vi "CO Serial CAL & Data Recording & DECADEv4.0.vi"() -> ()   [LabVIEW 2014]
uses:
  <vilib>/Platform/TimedLoop/XDataNode/timing_clust.ctl
  <vilib>/Platform/TimedLoop/XDataNode/nitl_modes.ctl
  <vilib>/Platform/TimedLoop/XDataNode/wakeup.ctl
  C:/Program Files (x86)/National Instruments/LabVIEW 2014/examples/Data Communication/Network Streams/Simple Network Streams/support/Network Stream Command.ctl
  <vilib>/Utility/error.llb/whitespace.ctl
  <vilib>/Instr/_visa.llb/VISA Configure Serial Port (Instr).vi
  <vilib>/Utility/tcp.llb/UDP Multicast Write-Only Open.vi
  <vilib>/platform/TimedLoop/XDataNode/XDataNode.xnode
  <vilib>/Platform/TimedLoop/XDataNode/XDNodeRunTimeDep.lvlib
panel:
  out "Stop File Write":bool
  out "Default file name":string
  in  "Flight Number 2":string="XXXX"
  out "status":bool
  out "CO Vacuum":bool
  out "CO CAL":bool
  out "error out":errorcluster
  out "CO Vacuum?":i16
  out "Control data":i32[](array[numeric])
  out "Control data out":string
  in  "VISA resource name":refnum<visa-resource-name>="ASRL8::INSTR"
  out "Serial VISA error":errorcluster
  out "SEPTIC TCP Error Out":errorcluster
  out "TCP packet\nSend To SEPTIC":bool
  in  "msec to wait":u32=330 caption="mSec to Wait"
  out "UDP Time Stamp Offset":i32=1
  out "Scan from String Error \nCounter from process loop":i32
  out "TCP Binary Packet":string
  in  "ue9LJ temp":u16
  out "FISH TCP Error Out":errorcluster
  out "TCP packet\nSend To FISH":bool
  out "UDP_Out_Error Out":errorcluster
  out "Data Array":string[](array[string])
  out "UDP_Out Status":bool
  out "Data Process Status":bool
  out "Command In":string[](array[string])
  out "ERR Counter":i32
  out "UDP_Out":string
  out "UDP_Pack_num":u32
  out "Flight Number":string
  out "OK RAW COUNTER":i32
  out "IN_CAL?":bool
  out "Redundent DATA":string
  out "Data String":string
  out "CO_Data_Buffer":string[](array[string])
  out "RAW DATA":string
  out "loop count":i32
  out "Number of Read error":i32
  out "Command In":string
  # "Pre-flight"
  # "CONC"
  # "SIG"
  # "SENS"
  # "ZERO"
  # "Lamp flow controller"
  # "Lamp temperature"
  # "Monochromater flow controller"
  # "Monochromater temperature"
  # "Monochromater pressure"
  # "Fluorescence cell pressure"
  # "Calibration gas pressure"
  # "Cell temperature"
  # "Calibration Concentration"
  # "ERROR number"
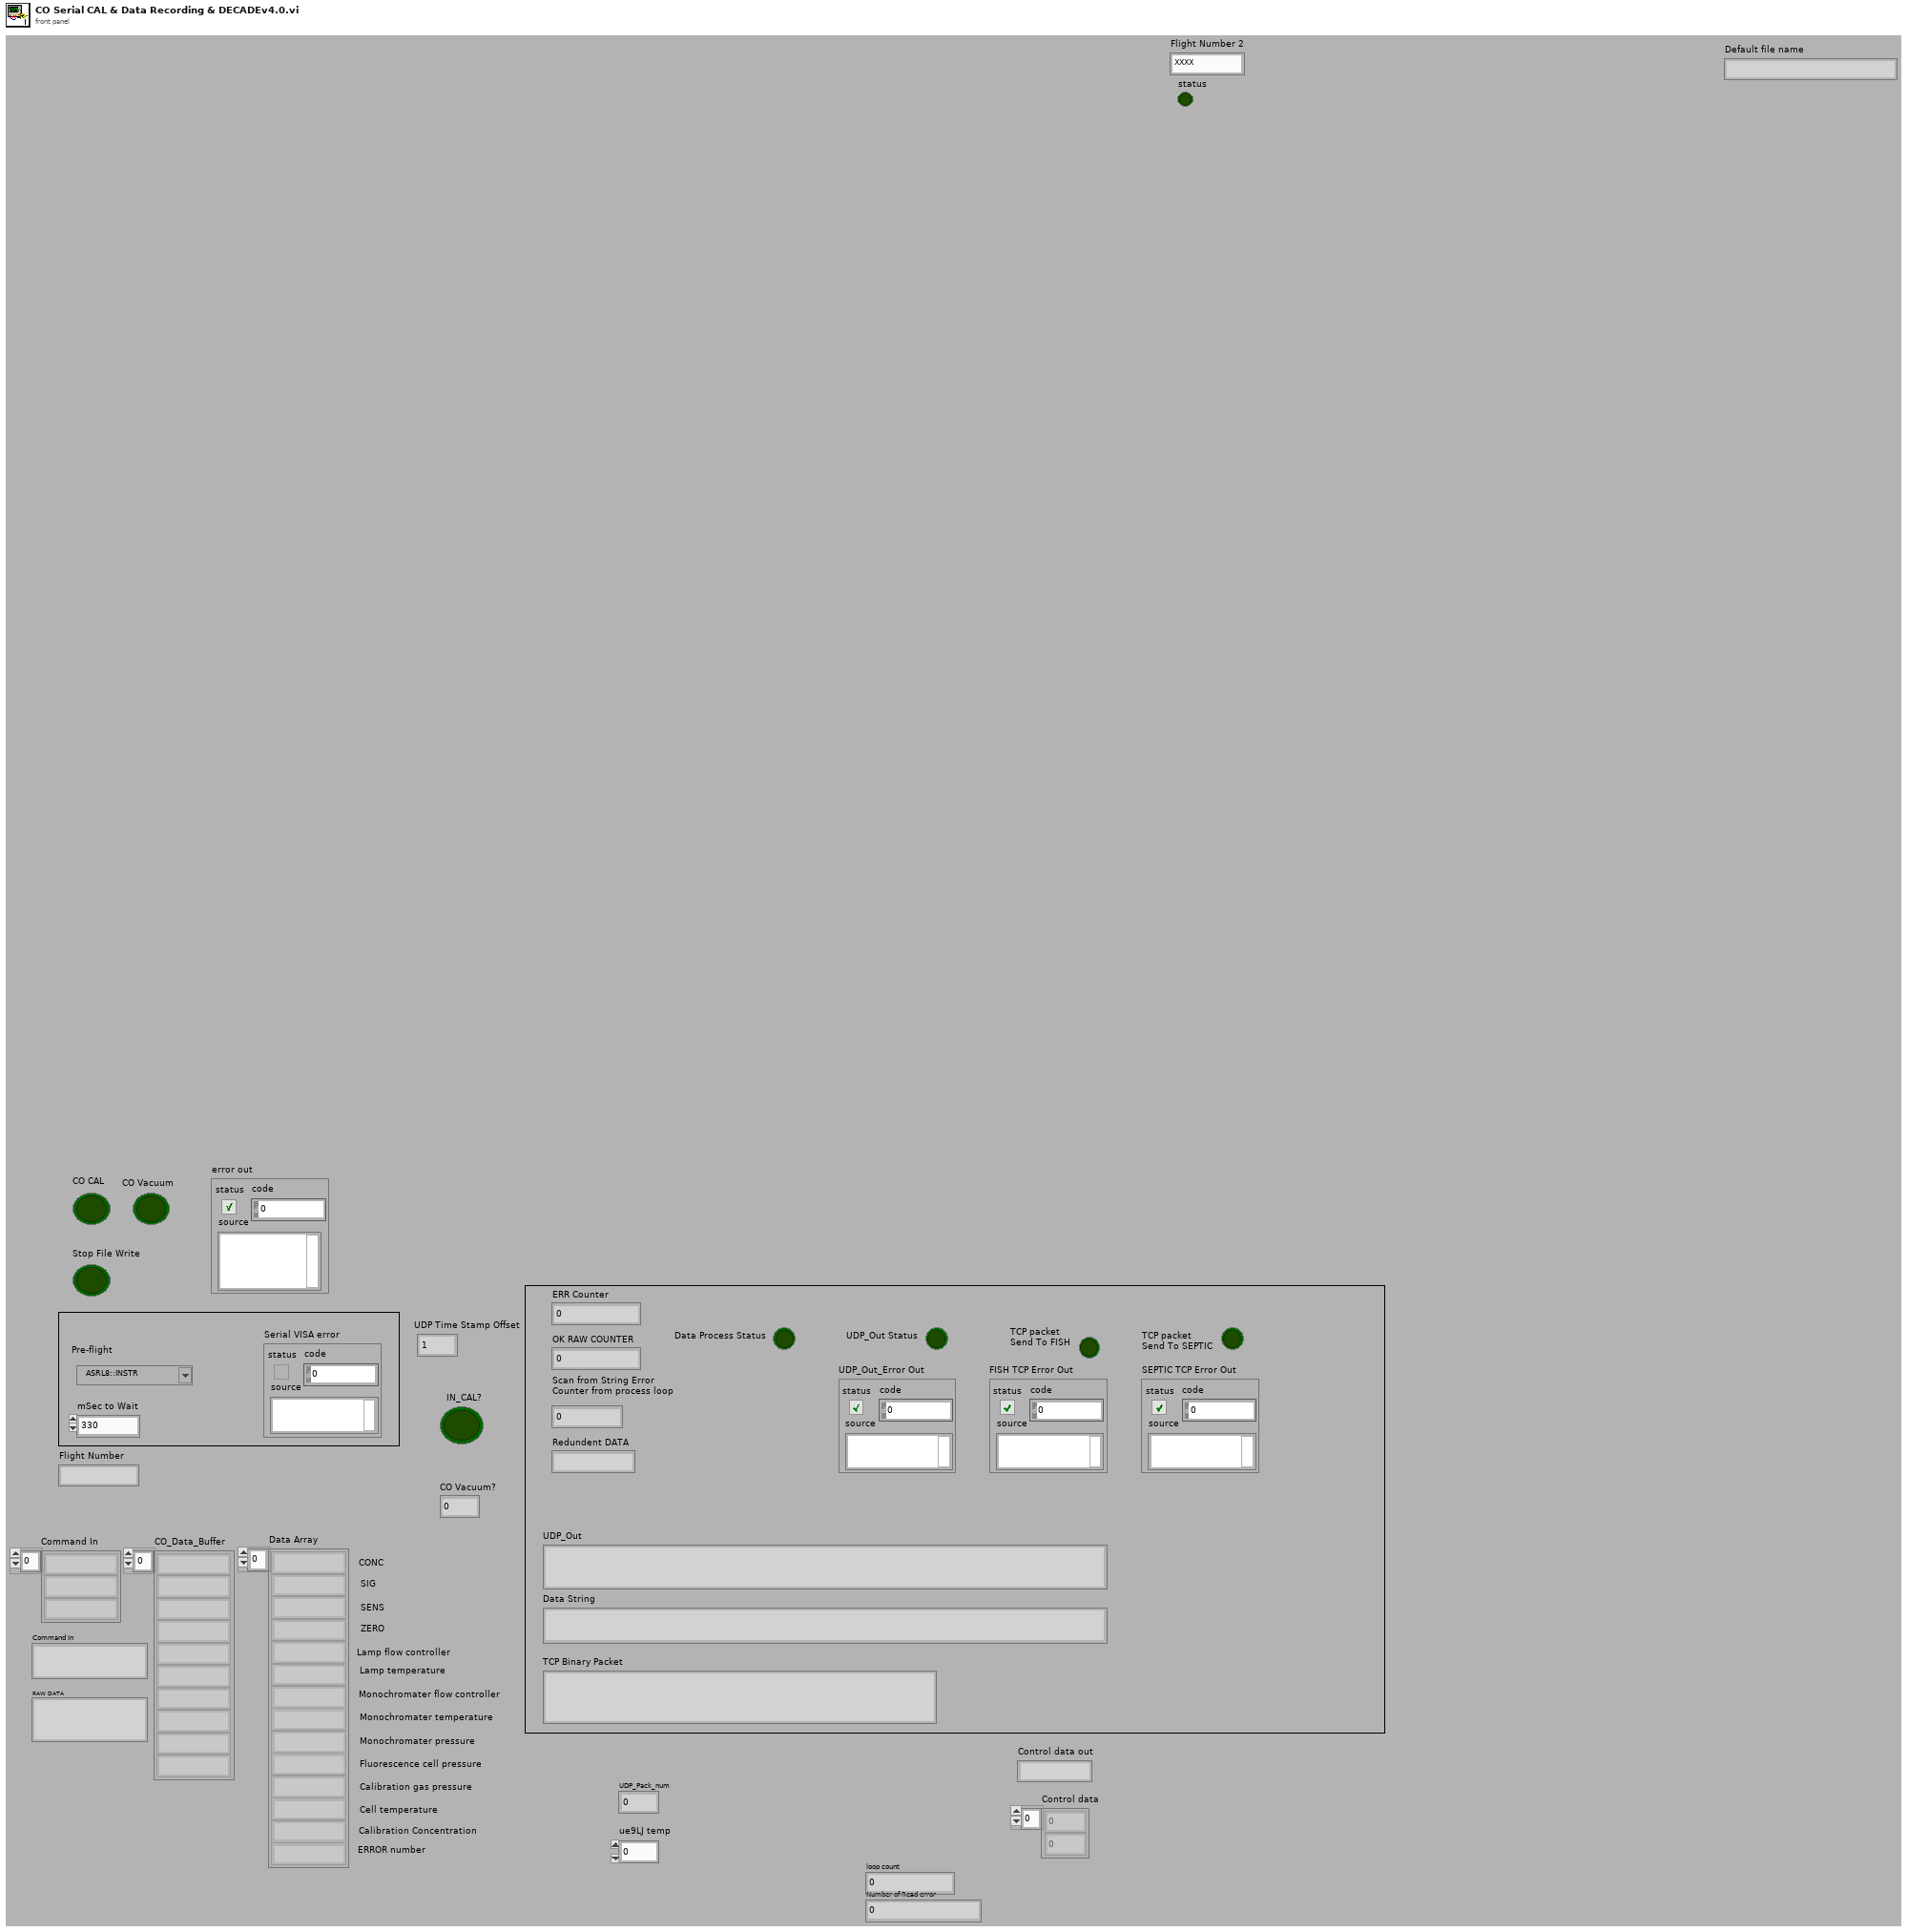
[diagram p1: front panel]
types:
  T1 = typedef "XDNodeRunTimeDep.lvlib/timing_clust.ctl" = cluster{"Expected End [f-1]":u64, "Actual End [f-1]":u64, "Finished Late? [f-1]":bool, "Expected End [i-1]":u64, "Actual End [i-1]":u64, "Finished Late? [i-1]":bool, "Expected Start [i]":u64, "Actual Start [i]":u64, "Expected Start [f]":u64, "Actual Start [f]":u64, "Source Name":string, "Structure Name":string, "Period":i64, "Deadline":i64, "Offset":i64, "Start":i64, "Priority":i32, "Timeout":i32, "Mode":T2, "Wakeup Reason":T3, "Error":errorcluster, "Source Type":string, "Secondary Source Type":string, "Global End Time":u64, "Global Start Time":u64, "Frame Duration":u64, "Iteration Duration":u64, "Assigned CPU":i32, "I/O Scan Engine Mode":u32}
  T2 = typedef "XDNodeRunTimeDep.lvlib/nitl_modes.ctl" = enum32{"No Change", "Process missed periods, maintain original phase", "Discard missed periods, maintain original phase", "Process missed periods, ignore original phase", "Discard missed periods, ignore original phase"}
  T3 = typedef "XDNodeRunTimeDep.lvlib/wakeup.ctl" = enum32{"Normal", "Aborted", "Asynchronous wakeup", "Timing source error", "Timed loop error", "Timeout"}
  T4 = typedef "Network Stream Command.ctl" = cluster{"Message":string, "Message Data":variant}
  T5 = enum16{"open", "replace", "create", "open or create", "replace or create", "replace or create with confirmation"}
  T6 = typedef "whitespace.ctl" = u16
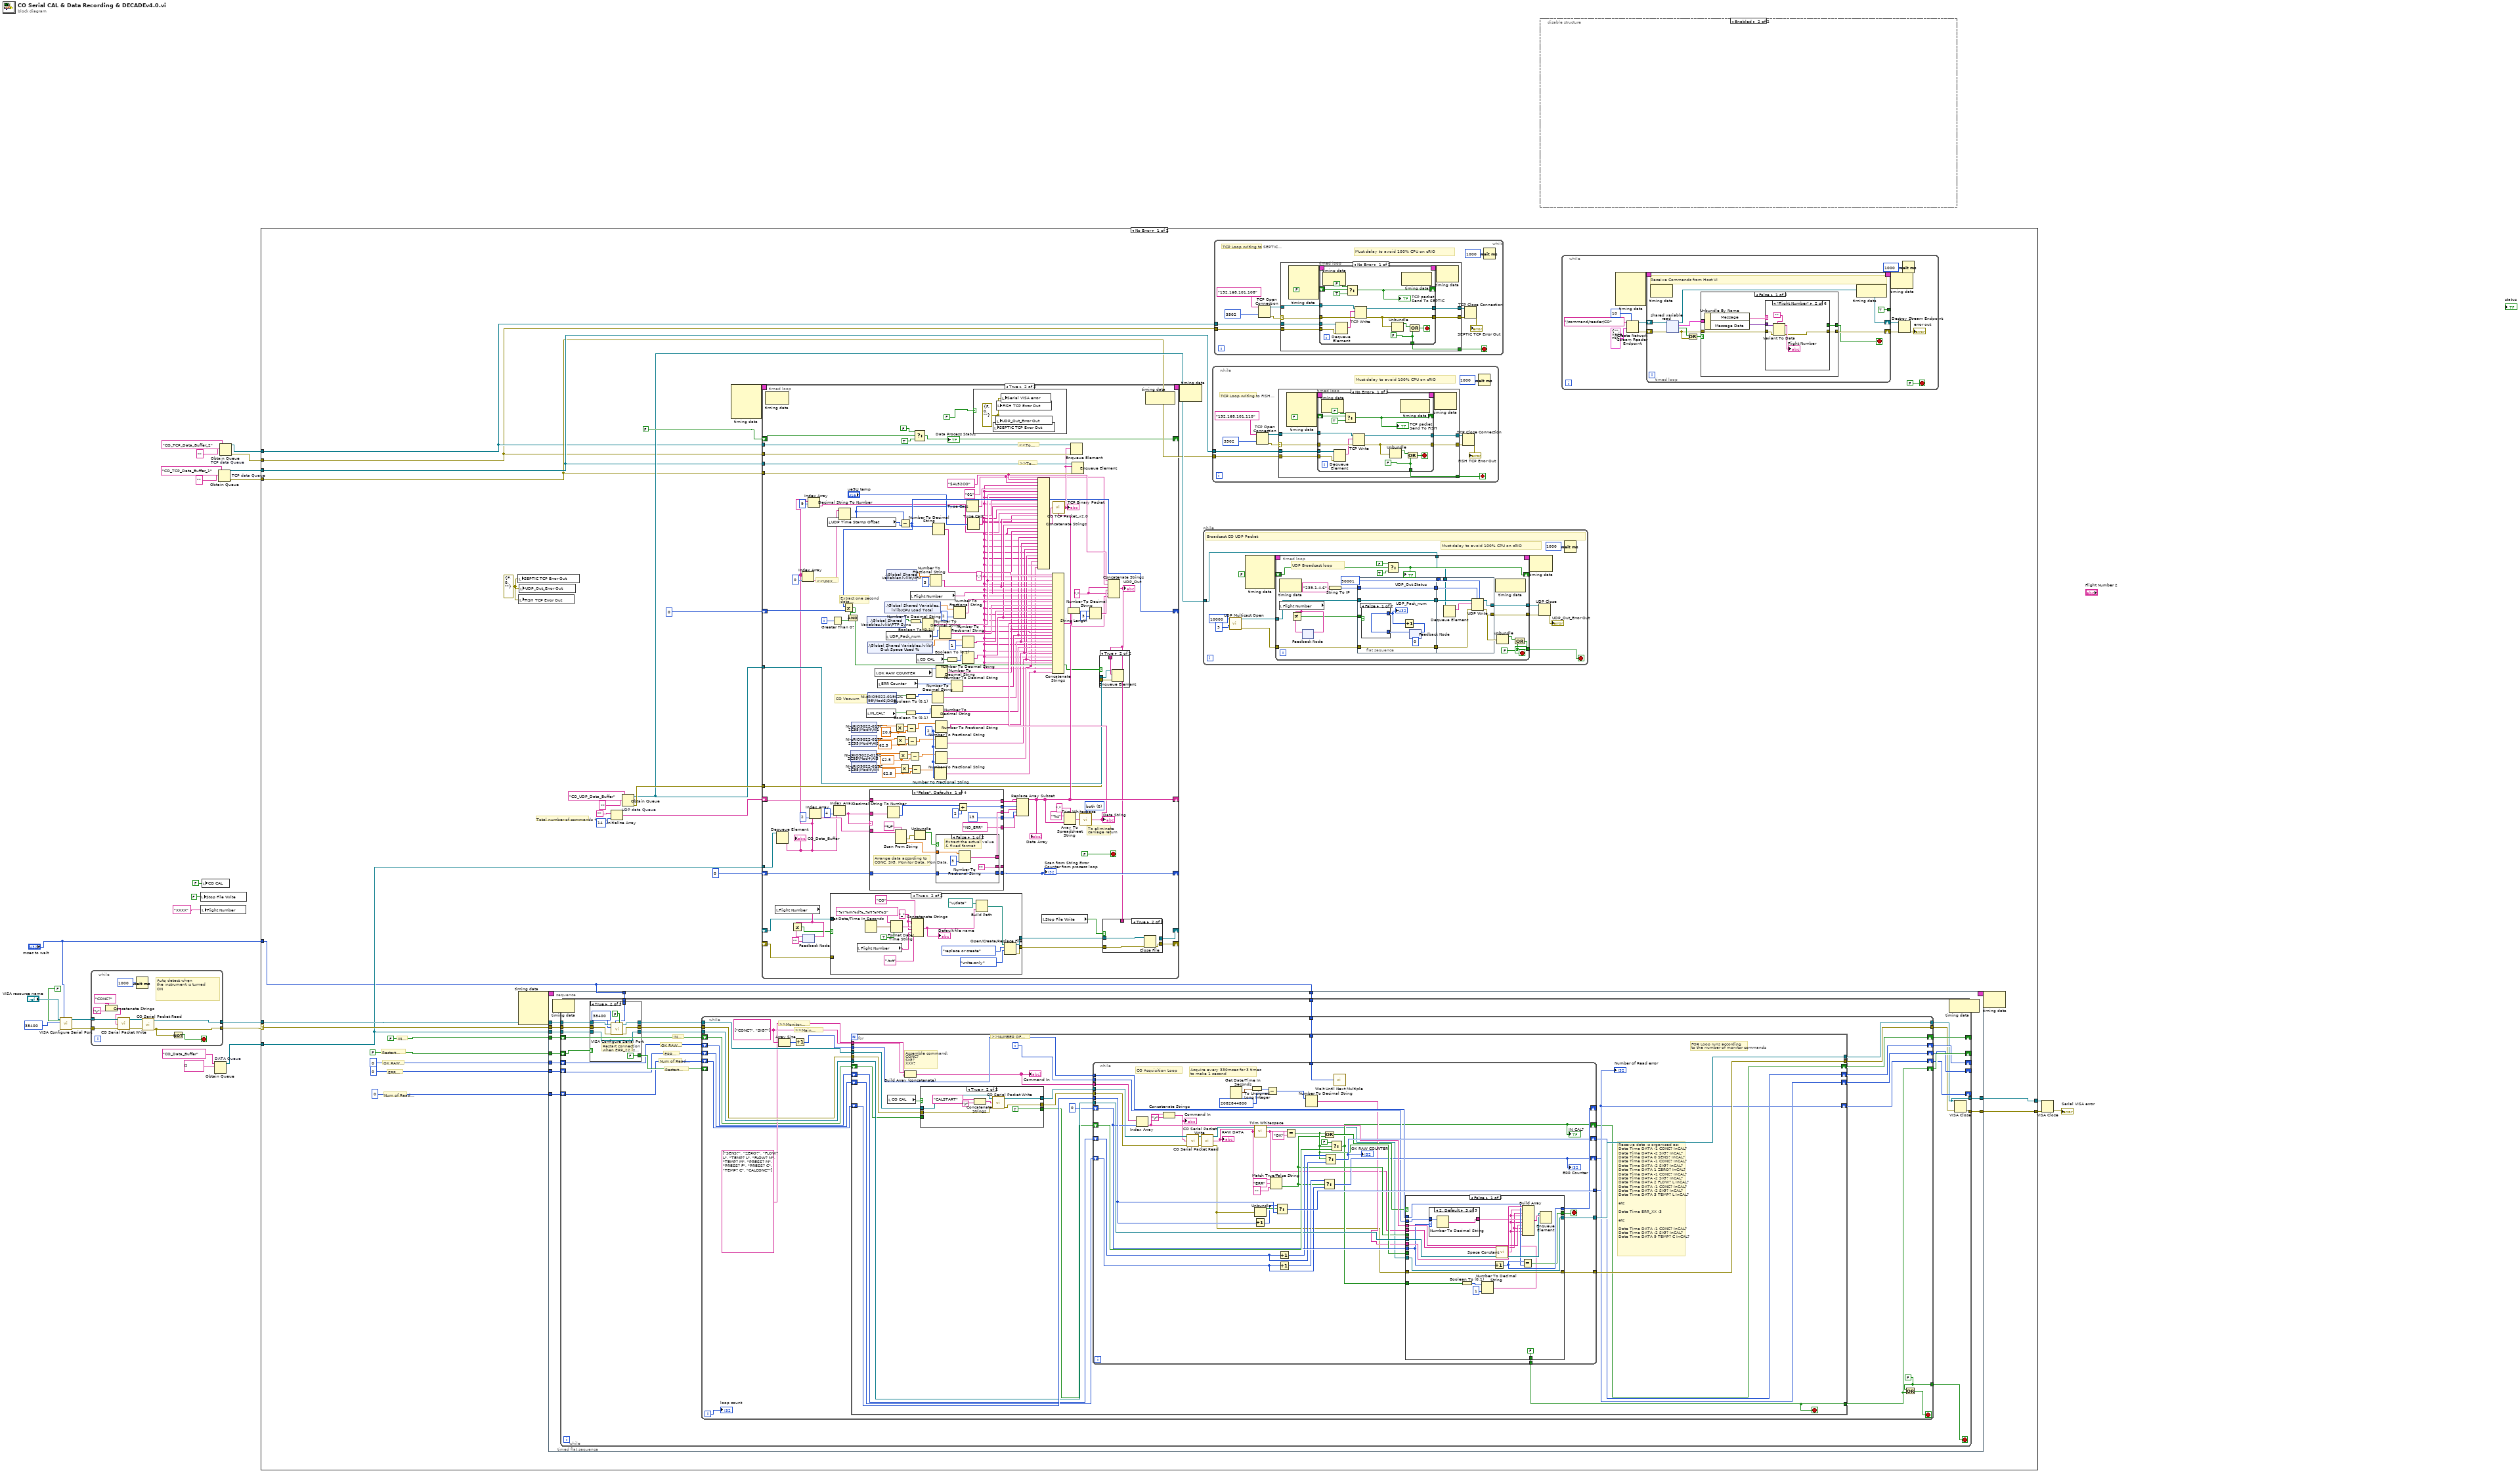
[diagram p0: block diagram]
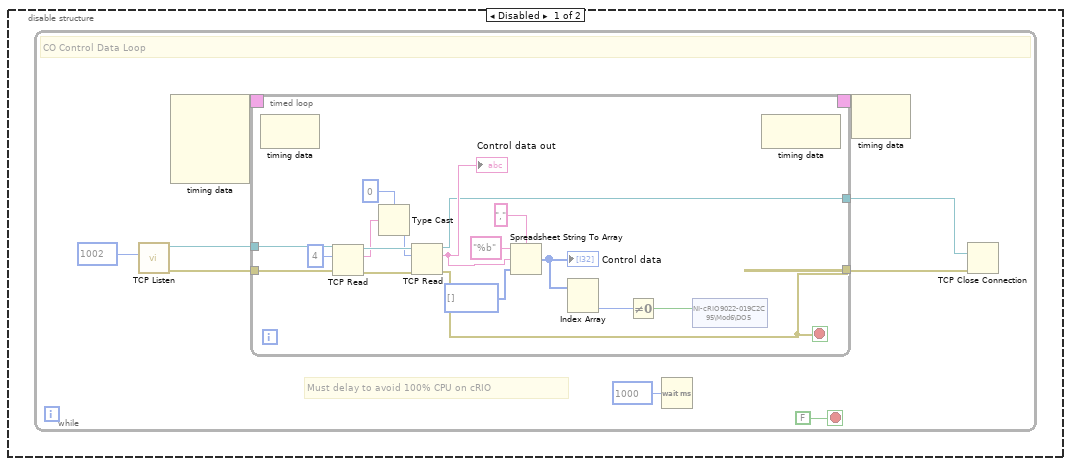
[diagram p2: hidden frame]
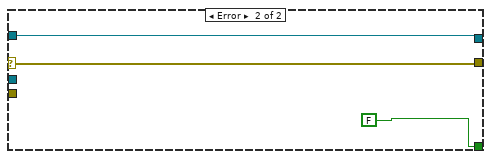
[diagram p3: hidden frame]
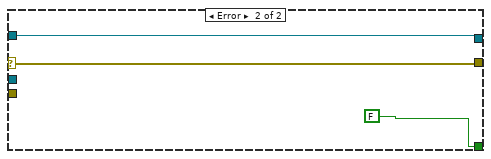
[diagram p4: hidden frame]
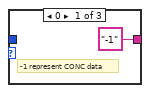
[diagram p6: hidden frame]
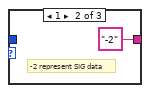
[diagram p7: hidden frame]
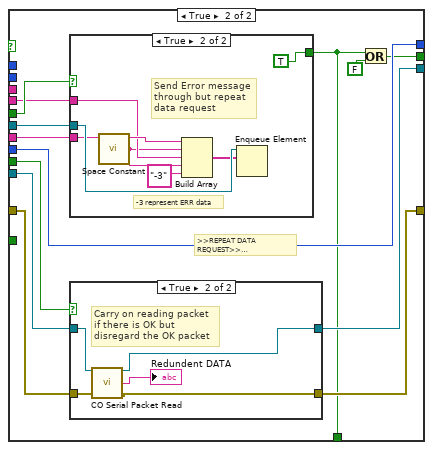
[diagram p8: hidden frame]
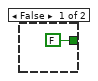
[diagram p10: hidden frame]
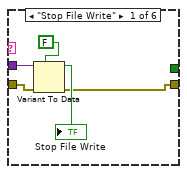
[diagram p12: hidden frame]
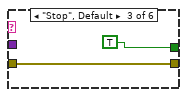
[diagram p13: hidden frame]
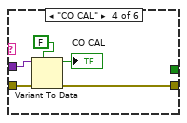
[diagram p14: hidden frame]
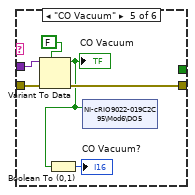
[diagram p15: hidden frame]
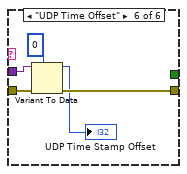
[diagram p16: hidden frame]
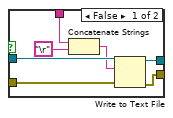
[diagram p19: hidden frame]
diagram:
  n1 = call-poly "VISA Configure Serial Port"("VISA resource name"="VISA resource name", "timeout (10sec)"="msec to wait", "Enable Termination\nChar (T)"=FALSE ("Enable Termination\nChar (T)"), "baud rate (9600)"=u32 38400) -> ("VISA resource name out"=w12:refnum<visa-resource-name>, "error out"=w11:errorcluster)  [unwired: 10 in]
  n2 = while {
    tunnel: w12 -> [w36]
    tunnel: w11 -> [w35]
    tunnel: [w29] -> w10
    tunnel: [w30] -> w9
    stop <- w34 stop-if-true
    # "Auto detect when\nthe instrument is turned \nON"
    n3 = Concatenate Strings("CONC?" ("Data in"), "\r") -> (w26:string)
    n4 = call "CO Serial Packet Write.vi"("VISA resource name In"=w36, "Data in"=w26, "error in (no error)"=w35) -> ("VISA resource name Out"=w32:refnum<visa-resource-name>, "error out"=w31:errorcluster)  [unwired: 11 in]
    n5 = Wait (ms)(milliseconds to wait=u32 1000) -> ()  [unwired: 1 out]
    n6 = call "CO Serial Packet Read.vi"("VISA resource In"=w32, "error in"=w31) -> ("VISA resource Out"=w29:refnum<visa-resource-name>, "error out"=w30:errorcluster)  [unwired: 11 in, 1 out]
    n7 = Not(x=w30) -> (.not. x?=w34:bool)
  }
  n8 = local write "Stop File Write"(FALSE ("Stop File Write")) -> ()
  n9 = local write "Flight Number"("XXXX" ("Flight Number")) -> ()
  n10 = local write "CO CAL"(FALSE ("CO CAL")) -> ()
  n11 = Obtain Queue "DATA Queue"(name (unnamed)="CO_Data_Buffer", element data type=string[] []) -> (queue out=w23:refnum<queue>)  [unwired: 3 in, 2 out]
  n12 = Obtain Queue "TCP data Queue"(name (unnamed)="CO_TCP_Data_Buffer_1", element data type="") -> (queue out=w22:refnum<queue>, error out=w21:errorcluster)  [unwired: 3 in, 1 out]
  n13 = Obtain Queue "TCP data Queue"(name (unnamed)="CO_TCP_Data_Buffer_2", element data type="") -> (queue out=w20:refnum<queue>, error out=w19:errorcluster)  [unwired: 3 in, 1 out]
  n14 = case shown="No Error" w9 {
    selector: w9 -> [w64 w717]
    tunnel: w10 -> [w65 w716]
    tunnel: [w66 w717] -> w15
    tunnel: [w42 w716] -> w14
    tunnel: w23 -> [w63 _]
    tunnel: w22 -> [w52 _]
    tunnel: w21 -> [w51 _]
    tunnel: w20 -> [w50 _]
    tunnel: w19 -> [w49 _]
    tunnel: "msec to wait" -> [w37 _]
    frame No Error {
      w48 = errorcluster {"status"=FALSE, "code"=0, "source"=""} ("UDP_Out_Error Out")
      # "Restart connection?"
      # "IN CAL?"
      # "OK RAW Counter"
      # "ERR Counter"
      # "Num of Read Error"
      # "Total number of commands + ERR"
      n15 = local write "SEPTIC TCP Error Out"(w48) -> ()
      n16 = node-c288() -> (w39:T1)  [unwired: 4 in]
      n17 = local write "FISH TCP Error Out"(w48) -> ()
      n18 = local write "UDP_Out_Error Out"(w48) -> ()
      n19 = timed-sequence {
        timing: w39 -> [_]
        timing-out: [_] -> w38
        tunnel: [w162] -> w66
        tunnel: w65 -> [w161]
        tunnel: w64 -> [w160]
        tunnel: w63 -> [w159]
        tunnel: FALSE -> [w158]
        tunnel: 0 -> [w157]
        tunnel: 0 -> [w156]
        tunnel: 0 -> [w155]
        tunnel: FALSE ("IN_CAL?") -> [w154]
        tunnel: [w153] -> w42
        tunnel: w37 -> [w152]
        tunnel: w37 -> [w151]
        n20 = timed-flat-sequence {
          tunnel: [w174] -> w162
          tunnel: w161 -> [w173]
          tunnel: w160 -> [w172]
          tunnel: w159 -> [w171]
          tunnel: w158 -> [w170]
          tunnel: w157 -> [w169]
          tunnel: w156 -> [w168]
          tunnel: w155 -> [w167]
          tunnel: w154 -> [w166]
          tunnel: [w165] -> w153
          tunnel: w152 -> [w164]
          tunnel: w151 -> [w163]
          n21 = node-c288() -> ()  [unwired: 1 in, 1 out]
          n22 = while {
            tunnel: [w179] -> w174
            tunnel: w173 -> [w196]
            tunnel: w172 -> [w195]
            tunnel: w171 -> [w193]
            shift-right: [w190] -> _
            shift-left: w170 -> [w191]
            shift-right: [w186] -> _
            shift-left: w169 -> [w187]
            shift-right: [w183] -> _
            shift-left: w168 -> [w185]
            shift-right: [w182] -> _
            shift-left: w167 -> [w184]
            shift-right: [w180] -> _
            shift-left: w166 -> [w181]
            tunnel: [w177] -> w165
            tunnel: w164 -> [w176]
            tunnel: w163 -> [w175]
            stop <- w189 stop-if-true
            # "Restart connection?"
            # "Num of Read Error"
            # "ERR Counter"
            # "IN CAL?"
            # "OK RAW Counter"
            n23 = case shown="True" w191 {
              selector: w191 -> [w198 _]
              tunnel: [w201 w207] -> w197
              tunnel: w196 -> [w201 w208]
              tunnel: [w200 w206] -> w194
              tunnel: w195 -> [w200 w205]
              tunnel: [w199 w210] -> w192
              tunnel: w193 -> [w199 w210]
              tunnel: [w198 FALSE] -> w188
              tunnel: w175 -> [_ w202]
              frame False {
              }
              frame True {
                # "Restart connection\nwhen ERR_22 is detected"
                n24 = call-poly "VISA Configure Serial Port"("VISA resource name"=w208, "timeout (10sec)"=w202, "Enable Termination\nChar (T)"=FALSE ("Enable Termination\nChar (T)"), "baud rate (9600)"=u32 38400, "error in (no error)"=w205) -> ("VISA resource name out"=w207:refnum<visa-resource-name>, "error out"=w206:errorcluster)  [unwired: 9 in]
              }
            }
            n25 = while {
              tunnel: [w232] -> w178
              tunnel: w197 -> [w231]
              tunnel: w194 -> [w230]
              tunnel: [w229] -> w177
              tunnel: w192 -> [w228]
              shift-right: [w219] -> w186
              shift-left: w187 -> [w223]
              shift-right: [w218] -> w183
              shift-left: w185 -> [w222]
              shift-right: [w217] -> w180
              shift-left: w181 -> [w221]
              shift-right: [w216] -> w182
              shift-left: w184 -> [w220]
              tunnel: [w212] -> w189
              shift-right: [w213] -> w190
              shift-left: w188 -> [_]
              tunnel: w176 -> [w211]
              i -> [w215]
              stop <- w214 stop-if-true
              w212 = FALSE
              w227 = string[] ["CONC?", "SIG?"]
              # ">>Main commands>>"
              # ">>Monitor Command>>"
              n26 = Array Size(array=w227) -> (size(s)=w224:i32)
              n27 = Increment(x=w224) -> (x+1=w226:i32)
              n28 = for {
                tunnel: w231 -> [w252]
                tunnel: w230 -> [w251]
                tunnel: [w257] -> w232
                shift-right: [w255] -> w216
                shift-left: w220 -> [w256]
                tunnel: [w254] -> w229
                tunnel: w228 -> [w253]
                tunnel: w226 -> [w247]
                shift-right: [w245] -> w217
                shift-left: w221 -> [w246]
                shift-right: [w243] -> w218
                shift-left: w222 -> [w244]
                shift-right: [w241] -> w219
                shift-left: w223 -> [w242]
                tunnel: string[] ["SENS?", "ZERO?", "FLOW? L", "TEMP? L", "FLOW? M", "TEMP? M", "PRESS? M", "PRESS? F", "PRESS? C", "TEMP? C", "CALCONC?"] -> [w238] mode=indexing
                tunnel: w227 -> [w239]
                tunnel: [w236] -> w213
                tunnel: w211 -> [w234]
                i -> [w237]
                stop <- w236 stop-if-true
                # "Receive data is organised as:\nDate Time DATA -1 CONC? InCAL?\nDate Time DATA -2 SIG? InCAL?\nDate Time DATA 0 SENS? InCAL?\nDate Time DATA -1 CONC? InCAL?\nDate Time DATA -2 SIG? InCAL?\nDate Time DATA 1 ZERO? InCAL?\nDate Time DATA -1 CONC? InCAL?\nDate Time DATA -2 SIG? InCAL?\nDate Time DATA 2 FLOW? L InCAL?\nDate Time DATA -1 CONC? InCAL?\nDate Time DATA -2 SIG? InCAL?\nDate Time DATA 3 TEMP? L InCAL?\n\netc\n\nDate Time ERR_XX -3\n\netc\n\nDate Time DATA -1 CONC? InCAL?\nDate Time DATA -2 SIG? InCAL?\nDate Time DATA 9 TEMP? C InCAL?"
                # "FOR Loop runs according\nto the number of monitor commands"
                # "Assemble command:\nCONC?\nSIG?\nXXX?"
                # ">>NUMBER OF COMMANDS>>"
                n29 = local read "CO CAL"() -> (w233:bool)
                n30 = Build Array (concatenate)(w239, w238) -> (w240:string[])
                "Command In" <- w240
                n31 = case shown="True" w233 {
                  tunnel: w252 -> [w357 w359]
                  tunnel: w251 -> [w356 w362]
                  tunnel: [w357 w360] -> w250
                  tunnel: [w356 w361] -> w249
                  tunnel: [w355 TRUE ("IN_CAL?")] -> w248
                  tunnel: w246 -> [w355 _]
                  frame False {
                  }
                  frame True {
                    n32 = Concatenate Strings("CALSTART" ("string"), "\r") -> (w358:string)
                    n33 = call "CO Serial Packet Write.vi"("VISA resource name In"=w359, "Data in"=w358, "error in (no error)"=w362) -> ("VISA resource name Out"=w360:refnum<visa-resource-name>, "error out"=w361:errorcluster)  [unwired: 11 in]
                  }
                }
                n34 = while {
                  tunnel: w249 -> [w264]
                  tunnel: [w291] -> w257
                  tunnel: w256 -> [w303]
                  tunnel: [w302] -> w255
                  tunnel: w240 -> [w295]
                  tunnel: [w292] -> w254
                  tunnel: w253 -> [w290]
                  tunnel: w250 -> [w266]
                  shift-right: [w267] -> w245
                  shift-left: w248 -> [w297]
                  shift-right: [w294] -> _
                  shift-left: 0 -> [w296]
                  tunnel: w247 -> [w287]
                  shift-right: [w284] -> w243
                  shift-left: w244 -> [w285]
                  shift-right: [w278] -> w241
                  shift-left: w242 -> [w280]
                  tunnel: w237 -> [w277]
                  tunnel: [w272] -> w236
                  tunnel: w234 -> [w258]
                  stop <- w293 stop-if-true
                  # "Acquire every 330msec for 3 times\nto make 1 second"
                  # "CO Acquisition Loop"
                  n35 = Index Array(array=w295, index=w296) -> (element=w289:string)
                  n36 = Concatenate Strings(w289, "\r") -> (w265:string)
                  "Command In" <- w265
                  n37 = call "CO Serial Packet Write.vi"("VISA resource name In"=w266, "Data in"=w265, "error in (no error)"=w264) -> ("VISA resource name Out"=w262:refnum<visa-resource-name>, "error out"=w263:errorcluster)  [unwired: 11 in]
                  n38 = call "CO Serial Packet Read.vi"("VISA resource In"=w262, "error in"=w263) -> ("VISA resource Out"=w261:refnum<visa-resource-name>, "Data Out"=w259:string, "error out"=w260:errorcluster)  [unwired: 11 in]
                  "RAW DATA" <- w259
                  n39 = Get Date/Time In Seconds() -> (seconds since 1Jan1904=w273:timestamp)
                  n40 = To Unsigned Long Integer(number=w273) -> (unsigned 32bit integer=w276:u32)
                  n41 = Increment(x=w303) -> (x+1=w299:i32)
                  n42 = call <vilib>:"Trim Whitespace.vi"("string"=w259) -> ("trimmed string"=w271:string)  [unwired: 1 in]
                  n43 = Unbundle(w260) -> ("status"=w300:bool)  [unwired: 2 out]
                  n44 = Subtract(x=w276, y=u32 2082844800) -> (x-y=w268:u32)
                  n45 = Match True/False String(2:"" ("false string"), 3:"ERR" ("true string"), 4:w259) -> (0:w279:bool)  [unwired: 1 out]
                  n46 = Select(t=w299, s=w300, f=w303) -> (s? t:f=w302:i32)
                  n47 = Increment(x=w285) -> (x+1=w286:i32)
                  n48 = Increment(x=w280) -> (x+1=w281:i32)
                  n49 = Equal?(x=w271, y="OK" ("string")) -> (x = y?=w282:bool)
                  n50 = Number To Decimal String(number=w268) -> (decimal integer string=w274:string)  [unwired: 1 in]
                  n51 = Select(t=w281, s=w279, f=w280) -> (s? t:f=w278:i32)
                  "ERR Counter" <- w278
                  n52 = Select(t=w286, s=w282, f=w285) -> (s? t:f=w284:i32)
                  "OK RAW COUNTER" <- w284
                  n53 = Compound Arithmetic op=OR(w282, w279) -> (w283:bool)
                  n54 = Select(t=FALSE, s=w282, f=w297) -> (s? t:f=w267:bool)
                  "IN_CAL?" <- w267
                  n55 = call "Wait Until Next Multiple"("Count(mSec)"=w258) -> ()  [unwired: 1 out]
                  n56 = case shown="False" w283 {
                    tunnel: w296 -> [w311 w339]
                    tunnel: [w322 w339] -> w294
                    tunnel: [w316 w329] -> w293
                    tunnel: w261 -> [w321 w338]
                    tunnel: w260 -> [w320 w337]
                    tunnel: [w321 w336] -> w292
                    tunnel: [w320 w335] -> w291
                    tunnel: w290 -> [w318 w333]
                    tunnel: w271 -> [w309 w331]
                    tunnel: w289 -> [w312 _]
                    tunnel: w274 -> [w317 w332]
                    tunnel: w279 -> [_ w334]
                    tunnel: w287 -> [w315 _]
                    tunnel: w282 -> [_ w330]
                    tunnel: w277 -> [w314 _]
                    tunnel: [FALSE w327] -> w272
                    tunnel: w267 -> [w308 _]
                    frame False {
                      n57 = case shown="2, Default" w311 {
                        tunnel: w314 -> [_ _ w326]
                        tunnel: ["-1" "-2" w325] -> w313
                        frame 0 {
                          # "-1 represent CONC data"
                        }
                        frame 1 {
                          # "-2 represent SIG data"
                        }
                        frame 2, Default {
                          n58 = Number To Decimal String(number=w326) -> (decimal integer string=w325:string)  [unwired: 1 in]
                        }
                      }
                      n59 = Boolean To (0,1)(Boolean=w308) -> (0, 1=w307:i16)
                      n60 = Number To Decimal String(number=w307, width (-)=i16 1) -> (decimal integer string=w304:string)
                      n61 = Increment(x=w311) -> (x+1=w322:i32)
                      n62 = call <vilib>:"Space Constant.vi"() -> ("String"=w305:string)
                      n63 = Equal?(x=w322, y=w315) -> (x = y?=w316:bool)
                      n64 = Build Array(w317, w305, w309, w305, w313, w305, w312, w309, w305, w304) -> (w319:string[])
                      n65 = Enqueue Element(queue=w318, element=w319) -> ()  [unwired: 2 in, 3 out]
                    }
                    frame True {
                      # ">>REPEAT DATA REQUEST>>\nif OK or ERR"
                      n66 = case shown="True" w334 {
                        tunnel: w333 -> [_ w354]
                        tunnel: w332 -> [_ w352]
                        tunnel: w331 -> [_ w351]
                        tunnel: [FALSE TRUE] -> w327
                        frame False {
                        }
                        frame True {
                          # "-3 represent ERR data"
                          # "Send Error message\nthrough but repeat\ndata request"
                          n67 = call <vilib>:"Space Constant.vi"() -> ("String"=w350:string)
                          n68 = Build Array(w352, w350, w351, w350, "-3" ("element")) -> (w353:string[])
                          n69 = Enqueue Element(queue=w354, element=w353) -> ()  [unwired: 2 in, 3 out]
                        }
                      }
                      n70 = case shown="True" w330 {
                        tunnel: w338 -> [w340 w345]
                        tunnel: w337 -> [w341 w346]
                        tunnel: [w340 w344] -> w336
                        tunnel: [w341 w342] -> w335
                        frame False {
                        }
                        frame True {
                          # "Carry on reading packet\nif there is OK but\ndisregard the OK packet"
                          n71 = call "CO Serial Packet Read.vi"("VISA resource In"=w345, "error in"=w346) -> ("VISA resource Out"=w344:refnum<visa-resource-name>, "Data Out"=→"Redundent DATA":string, "error out"=w342:errorcluster)  [unwired: 11 in]
                        }
                      }
                      n72 = Or(x=w327, y=FALSE) -> (x .or. y?=w329:bool)
                    }
                  }
                }
                "Number of Read error" <- w255
              }
              n73 = Or(x=w212, y=w213) -> (x .or. y?=w214:bool)
              "loop count" <- w215
            }
            n74 = VISA Close(VISA resource name=w177, error in (no error)=w178) -> (error out=w179:errorcluster)
          }
          n75 = node-c288() -> ()  [unwired: 1 in, 1 out]
        }
      }
      n76 = Initialize Array("", 14) -> (w60:string[])
      n77 = Obtain Queue "UDP data Queue"(name (unnamed)="CO_UDP_Data_Buffer", element data type="") -> (queue out=w55:refnum<queue>, error out=w56:errorcluster)  [unwired: 3 in, 1 out]
      n78 = node-c288() -> (w41:T1)  [unwired: 4 in]
      n79 = timed-loop {
        tunnel: w63 -> [w550]
        shift-right: [w525] -> _
        shift-left: w60 -> [w539]
        shift-right: [w526] -> _
        shift-left: FALSE -> [w529]
        tunnel: w52 -> [w524]
        tunnel: w51 -> [w523]
        tunnel: w55 -> [w521]
        tunnel: w56 -> [w520]
        shift-right: [w518] -> _
        shift-left: 0 -> [w519]
        shift-right: [w506] -> _
        shift-left: 0 -> [w512]
        tunnel: w50 -> [w510]
        tunnel: w49 -> [w509]
        timing: w41 -> [_]
        timing-out: [_] -> w40
        shift-right: [w497] -> _
        shift-left: _ -> [w490]
        shift-right: [w488] -> _
        shift-left: _ -> [w489]
        i -> [w515]
        stop <- FALSE stop-if-true
        w471 = 62.5 ("y")
        w472 = 62.5 ("y")
        w475 = 62.5 ("y")
        w478 = 20.0 ("y")
        w500 = i16 2 ("precision (6)")
        w531 = T6 0 items=["both", "start of string", "end of string"] ("location (both)")
        w435 = ","
        w450 = "01"
        w542 = ","
        w451 = "$AL52CO"
        # "CO Vacuum"
        # ">>To SEPTIC>>"
        # ">>To FISH>>"
        # "Extract one second data\nfor UDP sending"
        # ">>UNIX TIME>>"
        # "To eliminate\ncarriage return"
        n80 = node-c288() -> ()  [unwired: 1 in, 1 out]
        n81 = local read "Flight Number"() -> (w495:string)
        n82 = Dequeue Element(queue=w550) -> (element=w502:string[])  [unwired: 2 in, 3 out]
        "CO_Data_Buffer" <- w502
        n83 = Index Array(array=w502, index=0) -> (element=w513:string)
        n84 = feedback #1("" ("Flight Number")) -> (w494:string)
        n85 = Not Equal?(x=w495, y=w494) -> (x != y?=w493:bool)
        n86 = feedback-in #1(w495) -> ()
        n87 = Index Array(array=w502, index=9) -> (element=w444:string)
        n88 = Index Array(array=w502, index=2) -> (element=w537:string)
        n89 = local read "UDP Time Stamp Offset"() -> (w452:i32)
        n90 = case shown="True" w493 {
          tunnel: [w552 w554] -> w492
          tunnel: [w551 w553] -> w491
          tunnel: w490 -> [w552 _]
          tunnel: w489 -> [w551 _]
          frame False {
          }
          frame True {
            w561 = "_" ("string")
            n91 = local read "Flight Number"() -> (w567:string)
            n92 = Get Date/Time In Seconds() -> (seconds since 1Jan1904=w562:timestamp)
            n93 = Format Date/Time String(time format string (%c)="%Y%m%d%_%H%M%S", seconds (now)=w562, UTC format=TRUE) -> (date/time string=w565:string)
            n94 = Concatenate Strings("CO" ("string"), w561, w565, w561, w567, ".txt" ("string")) -> (w559:string)
            "Default file name" <- w559
            n95 = Build Path(base path=path "u:/data", name or relative path=w559) -> (appended path=w555:path)
            n96 = Open/Create/Replace File(file path (use dialog)=w555, operation (0:open)=T5."replace or create", access (0:read/write)=enum16{"read/write", "read-only", "write-only"}."write-only") -> (refnum out=w554:refnum<file>, error out=w553:errorcluster)  [unwired: 3 in, 1 out]
          }
        }
        n97 = Greater Than 0?(x=w515) -> (x > 0?=w514:bool)
        n98 = Index Array(array=w502, index=4) -> (element=w538:string)
        n99 = Decimal String To Number(string=w513) -> (number=w432:i32)  [unwired: 2 in, 1 out]
        n100 = shared-variable "NI-cRIO9022-019C2C95\\Mod4\\AI3"() -> (w470:dbl)  [unwired: 1 in, 1 out]
        n101 = shared-variable "NI-cRIO9022-019C2C95\\Mod4\\AI4"() -> (w468:dbl)  [unwired: 1 in, 1 out]
        n102 = shared-variable "NI-cRIO9022-019C2C95\\Mod4\\AI1"() -> (w480:dbl)  [unwired: 1 in, 1 out]
        n103 = shared-variable "NI-cRIO9022-019C2C95\\Mod4\\AI2"() -> (w474:dbl)  [unwired: 1 in, 1 out]
        n104 = local read "IN_CAL?"() -> (w457:bool)
        n105 = shared-variable ".\\Global Shared Variables.lvlib\\PTP Sync"() -> (w481:bool)  [unwired: 1 in, 1 out]
        n106 = shared-variable ".\\Global Shared Variables.lvlib\\Disk Space Used %"() -> (w461:dbl)  [unwired: 1 in, 1 out]
        n107 = shared-variable "NI-cRIO9022-019C2C95\\Mod6\\DO5"() -> (w454:bool)  [unwired: 1 in, 1 out]
        n108 = case shown="\"False\", Default" w538 {
          tunnel: w538 -> [w598 _ _ _]
          tunnel: w539 -> [w599 w621 w643 w657]
          tunnel: w537 -> [w590 w615 w637 w653]
          tunnel: [w599 w621 w643 w657] -> w536
          tunnel: [w596 0 ("index") 1 ("index") w654] -> w535
          tunnel: [w589 w611 w633 w653] -> w534
          tunnel: [w588 w612 w634 ""] -> _
          tunnel: w519 -> [w587 w614 w636 w655]
          tunnel: [w586 w613 w635 w655] -> w518
          tunnel: [13 ("index") 13 ("index") 13 ("index") w654] -> w505
          tunnel: ["NO_ERR" "NO_ERR" "NO_ERR" w653] -> w504
          frame "False", Default {
            # "Arrange data according to\nCONC, SIG, Monitor Data, Mon Data,"
            n109 = Decimal String To Number(string=w598) -> (number=w595:i32)  [unwired: 2 in, 1 out]
            n110 = Scan From String(format string="%f", input string=w590) -> (error out=w592:errorcluster, output 1=w593:dbl)  [unwired: 3 in, 2 out]
            n111 = Unbundle(w592) -> ("status"=w591:bool)  [unwired: 2 out]
            n112 = case shown="False" w591 {
              tunnel: [w604 ""] -> w589
              tunnel: w593 -> [w603 _]
              tunnel: w587 -> [w602 w607]
              tunnel: [w602 w606] -> w586
              tunnel: ["" "Scan from string error"] -> w588
              frame False {
                # "Extract the actual value\n& fixed format"
                n113 = Number To Fractional String(number=w603, precision (6)=i16 3) -> (F-format string=w604:string)  [unwired: 2 in]
              }
              frame True {
                # "If scan from string error,\nreplace data with empty\nstring"
                n114 = Increment(x=w607) -> (x+1=w606:i32)
              }
            }
            n115 = Add(x=w595, y=2) -> (x+y=w596:i32)
          }
          frame "-1" {
            # "Arrange data according to\nCONC, SIG, Monitor Data, Mon Data,"
            # "-1 represent CONC data"
            n116 = Scan From String(format string="%f", input string=w615) -> (error out=w617:errorcluster, output 1=w618:dbl)  [unwired: 3 in, 2 out]
            n117 = Unbundle(w617) -> ("status"=w616:bool)  [unwired: 2 out]
            n118 = case shown="False" w616 {
              tunnel: [w626 ""] -> w611
              tunnel: w618 -> [w625 _]
              tunnel: w614 -> [w624 w629]
              tunnel: [w624 w628] -> w613
              tunnel: ["" "Scan from string error"] -> w612
              frame False {
                # "Extract the actual value\n& fixed format"
                n119 = Number To Fractional String(number=w625, precision (6)=i16 5) -> (F-format string=w626:string)  [unwired: 2 in]
              }
              frame True {
                # "If scan from string error,\nreplace data with empty\nstring"
                n120 = Increment(x=w629) -> (x+1=w628:i32)
              }
            }
          }
          frame "-2" {
            # "Arrange data according to\nCONC, SIG, Monitor Data, Mon Data,"
            # "-2 represent SIG data"
            n121 = Scan From String(format string="%f", input string=w637) -> (error out=w639:errorcluster, output 1=w640:dbl)  [unwired: 3 in, 2 out]
            n122 = Unbundle(w639) -> ("status"=w638:bool)  [unwired: 2 out]
            n123 = case shown="False" w638 {
              tunnel: [w648 ""] -> w633
              tunnel: w640 -> [w647 _]
              tunnel: w636 -> [w646 w651]
              tunnel: [w646 w650] -> w635
              tunnel: ["" "Scan from string error"] -> w634
              frame False {
                # "Extract the actual value\n& fixed format"
                n124 = Number To Fractional String(number=w647, precision (6)=i16 3) -> (F-format string=w648:string)  [unwired: 2 in]
              }
              frame True {
                # "If scan from string error,\nreplace data with empty\nstring"
                n125 = Increment(x=w651) -> (x+1=w650:i32)
              }
            }
          }
          frame "-3" {
            w654 = 13 ("index")
            # "-3 represent ERR data"
          }
        }
        "Scan from String Error \nCounter from process loop" <- w518
        n126 = local read "OK RAW COUNTER"() -> (w540:i32)
        n127 = local read "ERR Counter"() -> (w499:i32)
        n128 = shared-variable ".\\Global Shared Variables.lvlib\\CPU Load Total"() -> (w486:dbl)  [unwired: 1 in, 1 out]
        n129 = local read "UDP_Pack_num"() -> (w546:u32)
        n130 = shared-variable ".\\Global Shared Variables.lvlib\\MFM"() -> (w485:dbl)  [unwired: 1 in, 1 out]
        n131 = Multiply(x=w480, y=w478) -> (x*y=w479:dbl)
        n132 = Multiply(x=w474, y=w475) -> (x*y=w476:dbl)
        n133 = Multiply(x=w470, y=w472) -> (x*y=w469:dbl)
        n134 = Multiply(x=w468, y=w471) -> (x*y=w467:dbl)
        n135 = Subtract(x=w432, y=w452) -> (x-y=w506:i32)
        n136 = Not Equal?(x=w506, y=w512) -> (x != y?=w516:bool)
        n137 = Compound Arithmetic op=AND(w516, w514) -> (w511:bool)
        n138 = Boolean To (0,1)(Boolean=w454) -> (0, 1=w453:i16)
        n139 = Boolean To (0,1)(Boolean=w457) -> (0, 1=w456:i16)
        n140 = Subtract(x=w479, y=w478) -> (x-y=w477:dbl)
        n141 = Subtract(x=w476, y=w475) -> (x-y=w473:dbl)
        n142 = Subtract(x=w469, y=w472) -> (x-y=w466:dbl)
        n143 = Boolean To (0,1)(Boolean=w481) -> (0, 1=w482:i16)
        n144 = local read "Flight Number"() -> (w445:string)
        n145 = Subtract(x=w467, y=w471) -> (x-y=w465:dbl)
        n146 = Select(t=FALSE, s=w529, f=TRUE) -> (s? t:f=w526:bool)
        "Data Process Status" <- w526
        n147 = local read "CO CAL"() -> (w459:bool)
        n148 = Number To Decimal String(number=w482) -> (decimal integer string=w448:string)  [unwired: 1 in]
        n149 = Number To Fractional String(number=w485, precision (6)=i16 3 ("width (-)")) -> (F-format string=w443:string)  [unwired: 2 in]
        n150 = Number To Decimal String(number=w456) -> (decimal integer string=w455:string)  [unwired: 1 in]
        n151 = Number To Decimal String(number=w453) -> (decimal integer string=w439:string)  [unwired: 1 in]
        n152 = Number To Decimal String(number=w506) -> (decimal integer string=w507:string)  [unwired: 1 in]
        n153 = Number To Fractional String(number=w465, precision (6)=w500) -> (F-format string=w434:string)  [unwired: 2 in]
        n154 = Number To Fractional String(number=w477, precision (6)=w500) -> (F-format string=w438:string)  [unwired: 2 in]
        n155 = Number To Fractional String(number=w473, precision (6)=w500) -> (F-format string=w437:string)  [unwired: 2 in]
        n156 = Number To Fractional String(number=w466, precision (6)=w500) -> (F-format string=w436:string)  [unwired: 2 in]
        n157 = Number To Decimal String(number=w540) -> (decimal integer string=w441:string)  [unwired: 1 in]
        n158 = Number To Decimal String(number=w546) -> (decimal integer string=w463:string)  [unwired: 1 in]
        n159 = Boolean To (0,1)(Boolean=w459) -> (0, 1=w460:i16)
        n160 = Number To Decimal String(number=w499) -> (decimal integer string=w440:string)  [unwired: 1 in]
        n161 = Number To Fractional String(number=w486, precision (6)=i16 2 ("width (-)")) -> (F-format string=w464:string)  [unwired: 2 in]
        n162 = Number To Fractional String(number=w461, precision (6)=i16 1 ("width (-)")) -> (F-format string=w458:string)  [unwired: 2 in]
        n163 = Number To Decimal String(number=w460) -> (decimal integer string=w442:string)  [unwired: 1 in]
        n164 = Type Cast(x=w432) -> (*(type *) &x=w449:string)  [unwired: 1 in]
        n165 = Type Cast(x="ue9LJ temp") -> (*(type *) &x=w446:string)  [unwired: 1 in]
        n166 = case shown="True" FALSE {
          frame False {
          }
          frame True {
            w580 = errorcluster {"status"=FALSE, "code"=0, "source"=""} ("UDP_Out_Error Out")
            n167 = local write "SEPTIC TCP Error Out"(w580) -> ()
            n168 = local write "UDP_Out_Error Out"(w580) -> ()
            n169 = local write "FISH TCP Error Out"(w580) -> ()
            n170 = local write "Serial VISA error"(w580) -> ()
          }
        }
        n171 = Replace Array Subset(array=w536, new element #1=w534, index #1=w535, new element #2=w504, index #2=w505) -> (w525:string[])
        "Data Array" <- w525
        n172 = Concatenate Strings(w451, w450, w435, w449, w435, w448, w435, w446, w435, w445, w435, w444, w435, w443, w435, w442, w435, w441, w435, w440, w435, w439, w435, w438, w435, w437, w435, w436, w435, w434) -> (w433:string)
        n173 = local read "Stop File Write"() -> (w496:bool)
        n174 = call "CO TCP Packet_v2.0.vi"("TCP Packet Content"=w433, "Data Array"=w525) -> ("TCP Binary Packet"=w508:string)  [unwired: 13 in]
        "TCP Binary Packet" <- w508
        n175 = Array To Spreadsheet String(delimiter (Tab)=",", array=w525, 3:"%s" ("format string")) -> (spreadsheet string=w530:string)
        n176 = Enqueue Element(queue=w510, element=w508, error in (no error)=w509) -> ()  [unwired: 1 in, 3 out]
        n177 = Enqueue Element(queue=w524, element=w508, error in (no error)=w523) -> ()  [unwired: 1 in, 3 out]
        n178 = call <vilib>:"Trim Whitespace.vi"("string"=w530, "location (both)"=w531) -> ("trimmed string"=w522:string)
        "Data String" <- w522
        n179 = Concatenate Strings(w507, w435, w448, w435, w443, w435, w445, w435, w464, w435, w463, w435, w458, w435, w442, w435, w522, w435, w441, w435, w440, w435, w439, w435, w455, w435, w438, w435, w437, w435, w436, w435, w434) -> (w541:string)
        n180 = String Length(string=w541) -> (length=w545:i32)
        n181 = Number To Decimal String(number=w545, width (-)=i16 3) -> (decimal integer string=w543:string)
        n182 = Concatenate Strings(w451, w450, w542, w543, w542, w541) -> (w498:string)
        "UDP_Out" <- w498
        n183 = case shown="True" w511 {
          tunnel: w498 -> [_ w583]
          tunnel: w521 -> [_ w582]
          tunnel: w520 -> [_ w581]
          frame False {
          }
          frame True {
            n184 = Enqueue Element(queue=w582, element=w583, error in (no error)=w581) -> ()  [unwired: 1 in, 3 out]
          }
        }
        n185 = case shown="True" w496 {
          tunnel: w498 -> [w572 _]
          tunnel: w492 -> [w574 w577]
          tunnel: w491 -> [w573 w576]
          tunnel: [w569 _] -> w497
          tunnel: [w568 w575] -> w488
          frame False {
            n186 = Concatenate Strings(w572, "\r") -> (w570:string)
            n187 = Write to Text File(file (use dialog)=w574, text=w570, error in=w573) -> (refnum out=w569:refnum<file>, error out=w568:errorcluster)  [unwired: 2 out]
          }
          frame True {
            n188 = Close File(refnum=w577, error in=w576) -> (error out=w575:errorcluster)  [unwired: 1 out]
          }
        }
        n189 = node-c288() -> ()  [unwired: 1 in, 1 out]
      }
      n190 = node-c288(w40) -> ()  [unwired: 1 out]
      n191 = while {
        tunnel: w55 -> [w661]
        stop <- w662 stop-if-true
        # "Must delay to avoid 100% CPU on cRIO"
        # "Broadcast CO UDP Packet"
        n192 = call-poly <vilib>:"UDP Multicast Open.vi"("time-to-live (1)"=u16 5, "port"=u16 10000) -> ("error out"=w669:errorcluster, "connection ID"=w670:refnum<k16>)  [unwired: 8 in]
        n193 = node-c288() -> (w672:T1)  [unwired: 4 in]
        n194 = timed-loop {
          tunnel: w670 -> [w692]
          tunnel: w669 -> [w691]
          timing: w672 -> [_]
          timing-out: [_] -> w671
          shift-right: [w679] -> _
          shift-left: FALSE -> [w682]
          tunnel: [w678] -> w664
          tunnel: [w676] -> w663
          tunnel: [w674] -> w662
          tunnel: w661 -> [w673]
          stop <- w675 stop-if-true
          w674 = FALSE
          # "UDP Broadcast loop"
          n195 = node-c288() -> ()  [unwired: 1 in, 1 out]
          n196 = local read "Flight Number"() -> (w685:string)
          n197 = feedback-in #2(w685) -> ()
          n198 = feedback #2() -> (w684:string)  [unwired: 1 in]
          n199 = Not Equal?(x=w685, y=w684) -> (x != y?=w683:bool)
          n200 = String To IP(1:"239.1.4.6" ("name")) -> (0:w689:u32)
          n201 = flat-sequence {
            tunnel: w689 -> [w699]
            tunnel: w691 -> [w700]
            tunnel: w692 -> [w701]
            tunnel: [w701] -> w688
            tunnel: [w700] -> w687
            tunnel: [w699] -> w686
            tunnel: w683 -> [w698]
            tunnel: u16 50001 ("port or service name") -> [w711]
            tunnel: w688 -> [w710]
            tunnel: w687 -> [w709]
            tunnel: w686 -> [w708]
            tunnel: [w707] -> w678
            tunnel: [w706] -> w676
            tunnel: w673 -> [w704]
            frame #0 {
              n202 = feedback #3(u32 0) -> (w695:u32)
              n203 = case shown="False" w698 {
                tunnel: w695 -> [w702 _]
                tunnel: [w702 u32 0] -> w694
                frame False {
                }
                frame True {
                }
              }
              "UDP_Pack_num" <- w694
              n204 = Increment(x=w694) -> (x+1=w696:u32)
              n205 = feedback-in #3(w696) -> ()
            }
            frame #1 {
              n206 = Dequeue Element(queue=w704) -> (element=w705:string)  [unwired: 2 in, 3 out]
              n207 = UDP Write(address=w708, port or service name=w711, connection ID=w710, data in=w705, 8:w709) -> (error out=w706:errorcluster, 3:w707:refnum<k16>)  [unwired: 1 in]
            }
          }
          n208 = Select(t=FALSE, s=w682, f=TRUE) -> (s? t:f=w679:bool)
          "UDP_Out Status" <- w679
          n209 = node-c288() -> ()  [unwired: 1 in, 1 out]
          n210 = Unbundle(w676) -> ("status"=w677:bool)  [unwired: 2 out]
          n211 = Compound Arithmetic op=OR(w677, w674) -> (w675:bool)
        }
        n212 = node-c288(w671) -> ()  [unwired: 1 out]
        n213 = UDP Close(connection ID=w664, 8:w663) -> (error out=→"UDP_Out_Error Out":errorcluster)  [unwired: 1 out]
        n214 = Wait (ms)(milliseconds to wait=u32 1000) -> ()  [unwired: 1 out]
      }
      n215 = while {
        tunnel: w52 -> [w111]
        tunnel: w51 -> [w110]
        stop <- w114 stop-if-true
        # "Must delay to avoid 100% CPU on cRIO"
        # "TCP Loop writing to FISH Tank"
        n216 = TCP Open Connection(address="192.168.101.110", remote port or service name=u16 3502) -> (connection ID=w117:refnum<k5>, error out=w112:errorcluster)  [unwired: 3 in]
        n217 = case shown="No Error" w112 {
          selector: w112 -> [w122 w149]
          tunnel: w117 -> [w127 w150]
          tunnel: [w126 w150] -> w116
          tunnel: [w125 w149] -> w115
          tunnel: [w124 FALSE] -> w114
          tunnel: w111 -> [w121 _]
          tunnel: w110 -> [w120 _]
          frame No Error {
            n218 = node-c288() -> (w129:T1)  [unwired: 4 in]
            n219 = timed-loop {
              tunnel: w127 -> [w143]
              tunnel: w122 -> [w142]
              tunnel: [w141] -> w126
              tunnel: [w140] -> w125
              tunnel: [w130] -> w124
              shift-right: [w134] -> _
              shift-left: FALSE -> [w137]
              timing: w129 -> [_]
              timing-out: [_] -> w128
              tunnel: w121 -> [w133]
              tunnel: w120 -> [w132]
              stop <- w138 stop-if-true
              w130 = FALSE
              n220 = node-c288() -> ()  [unwired: 1 in, 1 out]
              n221 = Dequeue Element(queue=w133, error in (no error)=w132) -> (element=w131:string)  [unwired: 1 in, 3 out]
              n222 = Select(t=FALSE, s=w137, f=TRUE) -> (s? t:f=w134:bool)
              "TCP packet\nSend To FISH" <- w134
              n223 = TCP Write(connection ID=w143, data in=w131, error in (no error)=w142) -> (connection ID out=w141:refnum<k5>, error out=w140:errorcluster)  [unwired: 1 in, 1 out]
              n224 = Unbundle(w140) -> ("status"=w139:bool)  [unwired: 2 out]
              n225 = node-c288() -> ()  [unwired: 1 in, 1 out]
              n226 = Compound Arithmetic op=OR(w139, w130) -> (w138:bool)
            }
            n227 = node-c288(w128) -> ()  [unwired: 1 out]
          }
          frame Error {
          }
        }
        n228 = TCP Close Connection(connection ID=w116, error in (no error)=w115) -> (error out=→"FISH TCP Error Out":errorcluster)  [unwired: 1 in, 1 out]
        n229 = Wait (ms)(milliseconds to wait=u32 1000) -> ()  [unwired: 1 out]
      }
      n230 = while {
        tunnel: w50 -> [w69]
        tunnel: w49 -> [w68]
        stop <- w72 stop-if-true
        # "Must delay to avoid 100% CPU on cRIO"
        # "TCP Loop writing to SEPTIC Tank"
        n231 = TCP Open Connection(address="192.168.101.108", remote port or service name=u16 3502) -> (connection ID=w75:refnum<k5>, error out=w70:errorcluster)  [unwired: 3 in]
        n232 = case shown="No Error" w70 {
          selector: w70 -> [w80 w107]
          tunnel: w75 -> [w85 w108]
          tunnel: [w84 w108] -> w74
          tunnel: [w83 w107] -> w73
          tunnel: [w82 FALSE] -> w72
          tunnel: w69 -> [w79 _]
          tunnel: w68 -> [w78 _]
          frame No Error {
            n233 = node-c288() -> (w87:T1)  [unwired: 4 in]
            n234 = timed-loop {
              tunnel: w85 -> [w101]
              tunnel: w80 -> [w100]
              tunnel: [w99] -> w84
              tunnel: [w98] -> w83
              tunnel: [w88] -> w82
              shift-right: [w92] -> _
              shift-left: FALSE -> [w95]
              timing: w87 -> [_]
              timing-out: [_] -> w86
              tunnel: w79 -> [w91]
              tunnel: w78 -> [w90]
              stop <- w96 stop-if-true
              w88 = FALSE
              n235 = node-c288() -> ()  [unwired: 1 in, 1 out]
              n236 = Dequeue Element(queue=w91, error in (no error)=w90) -> (element=w89:string)  [unwired: 1 in, 3 out]
              n237 = Select(t=FALSE, s=w95, f=TRUE) -> (s? t:f=w92:bool)
              "TCP packet\nSend To SEPTIC" <- w92
              n238 = TCP Write(connection ID=w101, data in=w89, error in (no error)=w100) -> (connection ID out=w99:refnum<k5>, error out=w98:errorcluster)  [unwired: 1 in, 1 out]
              n239 = Unbundle(w98) -> ("status"=w97:bool)  [unwired: 2 out]
              n240 = node-c288() -> ()  [unwired: 1 in, 1 out]
              n241 = Compound Arithmetic op=OR(w97, w88) -> (w96:bool)
            }
            n242 = node-c288(w86) -> ()  [unwired: 1 out]
          }
          frame Error {
          }
        }
        n243 = TCP Close Connection(connection ID=w74, error in (no error)=w73) -> (error out=→"SEPTIC TCP Error Out":errorcluster)  [unwired: 1 in, 1 out]
        n244 = Wait (ms)(milliseconds to wait=u32 1000) -> ()  [unwired: 1 out]
      }
      n245 = while {
        stop <- FALSE stop-if-true
        n246 = node-c288() -> (w371:T1)  [unwired: 4 in]
        n247 = Create Network Stream Reader Endpoint(7:10 ("reader buffer size"), 9:T4 {"Message"="", "Message Data"=variant} ("Message Cluster"), 11:"/command/reader/CO" ("reader url")) -> (0:w377:errorcluster, 3:w378:refnum<k21>)  [unwired: 4 in]
        n248 = timed-loop "Host->Target Command Reader" {
          shift-right: [w388] -> w375
          shift-left: w377 -> [w391]
          shift-right: [w389] -> w374
          shift-left: w378 -> [w390]
          tunnel: [TRUE] -> _
          timing: w371 -> [_]
          timing-out: [_] -> w370
          stop <- w382 stop-if-true
          # "Receive Commands from Host VI"
          n249 = node-c288() -> ()  [unwired: 1 in, 1 out]
          n250 = shared-variable-read(w390, w391) -> (w389:refnum<k21>, w384:errorcluster, w386:bool, w387:T4)  [unwired: 1 in]
          n251 = Or(x=w386, y=w384) -> (x .or. y?=w385:bool)
          n252 = case shown="False" w385 {
            selector: w385 -> [_ w428]
            tunnel: w384 -> [w399 w429]
            tunnel: [w398 w429] -> w388
            tunnel: w387 -> [w397 _]
            tunnel: [w394 w428] -> w382
            frame False {
              n253 = Unbundle By Name(w397) -> ("Message"=w396:string, "Message Data"=w395:variant)
              n254 = case shown="\"Flight Number\"" w396 {
                tunnel: w399 -> [w403 w408 w410 w416 w422 w427]
                tunnel: [w400 w405 w410 w415 w421 w426] -> w398
                tunnel: w395 -> [w404 w409 _ w414 w420 w425]
                tunnel: [_ _ TRUE _ _ _] -> w394
                frame "Stop File Write" {
                  n255 = Variant To Data(error in=w403, type=FALSE, Variant=w404) -> (data=→"Stop File Write":bool, error out=w400:errorcluster)
                }
                frame "Flight Number" {
                  n256 = Variant To Data(error in=w408, type="", Variant=w409) -> (data=→"Flight Number":string, error out=w405:errorcluster)
                }
                frame "Stop", Default {
                }
                frame "CO CAL" {
                  n257 = Variant To Data(error in=w416, type=FALSE, Variant=w414) -> (data=→"CO CAL":bool, error out=w415:errorcluster)
                }
                frame "CO Vacuum" {
                  n258 = Variant To Data(error in=w422, type=FALSE, Variant=w420) -> (data=w417:bool, error out=w421:errorcluster)
                  "CO Vacuum" <- w417
                  n259 = Boolean To (0,1)(Boolean=w417) -> (0, 1=→"CO Vacuum?":i16)
                  n260 = shared-variable "NI-cRIO9022-019C2C95\\Mod6\\DO5"(w417) -> ()  [unwired: 1 in, 1 out]
                }
                frame "UDP Time Offset" {
                  n261 = Variant To Data(error in=w427, type=0, Variant=w425) -> (data=→"UDP Time Stamp Offset":i32, error out=w426:errorcluster)
                }
              }
            }
            frame True {
            }
          }
          n262 = node-c288() -> ()  [unwired: 1 in, 1 out]
        }
        n263 = node-c288(w370) -> ()  [unwired: 1 out]
        n264 = Destroy Stream Endpoint(8:w375, 11:w374) -> (0:→"error out":errorcluster)
        n265 = Wait (ms)(milliseconds to wait=u32 1000) -> ()  [unwired: 1 out]
      }
      n266 = node-c288(w38) -> ()  [unwired: 1 out]
    }
    frame Error {
    }
  }
  n267 = disable-structure shown="Enabled" {
    frame Disabled {
      n268 = while {
        stop <- FALSE stop-if-true
        # "Must delay to avoid 100% CPU on cRIO"
        # "CO Control Data Loop"
        n269 = call <vilib>:"TCP Listen.vi"("port"=u16 1002) -> ("error out"=w722:errorcluster, "connection ID"=w723:refnum<k5>)  [unwired: 6 in, 3 out]
        n270 = node-c288() -> (w726:T1)  [unwired: 4 in]
        n271 = timed-loop {
          timing: w726 -> [_]
          timing-out: [_] -> w725
          tunnel: w723 -> [w743]
          tunnel: w722 -> [w742]
          tunnel: [w732] -> w721
          tunnel: [w731] -> w720
          stop <- w731 stop-if-true
          n272 = node-c288() -> ()  [unwired: 1 in, 1 out]
          n273 = TCP Read(connection ID=w743, bytes to read=4, error in (no error)=w742) -> (connection ID out=w740:refnum<k5>, data out=w737:string, error out=w739:errorcluster)  [unwired: 2 in]
          n274 = Type Cast(type=0, x=w737) -> (*(type *) &x=w736:i32)
          n275 = TCP Read(connection ID=w740, bytes to read=w736, error in (no error)=w739) -> (connection ID out=w732:refnum<k5>, data out=w733:string, error out=w731:errorcluster)  [unwired: 2 in]
          "Control data out" <- w733
          n276 = Spreadsheet String To Array(delimiter (Tab)=",", format string="%b", spreadsheet string=w733, array type (2D Dbl)=i32[] []) -> (array=w730:i32[])
          "Control data" <- w730
          n277 = Index Array(array=w730) -> (element #2=w728:i32)  [unwired: 2 in, 1 out]
          n278 = Not Equal To 0?(x=w728) -> (x != 0?=w727:bool)
          n279 = shared-variable "NI-cRIO9022-019C2C95\\Mod6\\DO5"(w727) -> ()  [unwired: 1 in, 1 out]
          n280 = node-c288() -> ()  [unwired: 1 in, 1 out]
        }
        n281 = Wait (ms)(milliseconds to wait=u32 1000) -> ()  [unwired: 1 out]
        n282 = node-c288(w725) -> ()  [unwired: 1 out]
        n283 = TCP Close Connection(connection ID=w721, error in (no error)=w720) -> ()  [unwired: 1 in, 2 out]
      }
    }
    frame Enabled {
    }
  }
  n284 = VISA Close(VISA resource name=w14, error in (no error)=w15) -> (error out=→"Serial VISA error":errorcluster)
